vi "DT_Triangulation Main.vi"(11 "Points In":cluster{"x":dbl, "y":dbl, "index":i32}[](array[cluster])) -> (0 "error":i32, 2 "Triangles":i32[][](array[numeric]), 3 "Points Out":cluster{"x":dbl, "y":dbl, "index":i32}[](array[cluster]))   [LabVIEW 2020, in "NI_AAL_Geometry.lvlib"]
uses:
  <vilib>/Analysis/NI_AAL_Geometry.lvlib
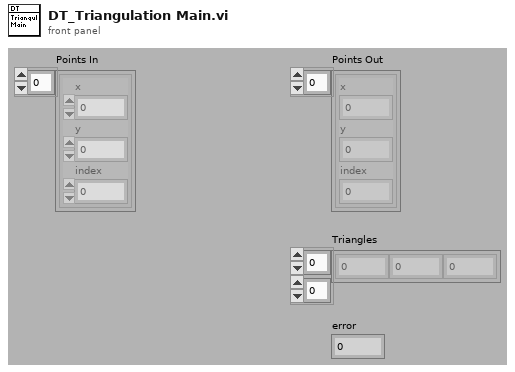
[diagram p1: front panel]
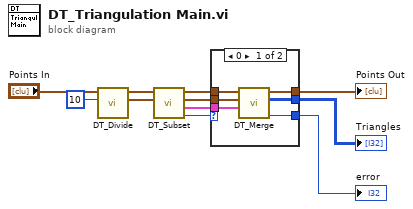
[diagram p0: block diagram]
diagram:
  n1 = call <vilib>:"DT_Divide.vi"("min subset size"=10, "Points In"="Points In") -> ("Subset"=w7:cluster{"start idx":i32, "length":i32}[], "Points Out"=w5:cluster{"x":dbl, "y":dbl, "index":i32}[])  [unwired: 8 out]
  n2 = call <vilib>:"DT_Subset.vi"("Subset"=w7, "Points In"=w5) -> ("error"=w2:i32, "Subset Triangles"=w6:cluster{"Triangles":i32[][]}[], "Subset Out"=w3:cluster{"start idx":i32, "length":i32}[], "Points Out"=w4:cluster{"x":dbl, "y":dbl, "index":i32}[])  [unwired: 6 out]
  n3 = case shown="0" w2 {
    selector: w2 -> [_ w18]
    tunnel: [w17 w19] -> w10
    tunnel: [w16 _] -> w8
    tunnel: w6 -> [w15 _]
    tunnel: w4 -> [w14 w19]
    tunnel: w3 -> [w13 _]
    tunnel: [w12 w18] -> w1
    frame 0 {
      n4 = call <vilib>:"DT_Merge.vi"("Subset Triangles"=w15, "Subset"=w13, "Points In"=w14) -> ("error"=w12:i32, "Triangles"=w16:i32[][], "Points Out"=w17:cluster{"x":dbl, "y":dbl, "index":i32}[])  [unwired: 1 in, 5 out]
    }
    frame Default {
    }
  }
  "Triangles" <- w8
  "Points Out" <- w10
  "error" <- w1
